vi "TeardownBeforeStart.vi"(6 "Error":errorcluster, 7 "ConcreteActor":refnum<class "ConcreteActor.lvclass">, 11 "UnheardMessages":refnum<class "Message.lvclass">[](array[class])) -> (5 "ConcreteActor":refnum<class "ConcreteActor.lvclass">)   [LabVIEW 2020, in "_Template.lvlib" / "ActorTemplate.lvlib" / "{{Name}}.lvlib" / "ConcreteActor.lvclass"]
uses:
  ConcreteActor.lvclass
  ConcreteActor.lvclass/ConcreteActor.ctl
  jettl/jettl/Actor/Actor.lvclass
  jettl/jettl/Message/Message.lvclass
panel:
  # "This front panel should not be manipulated."
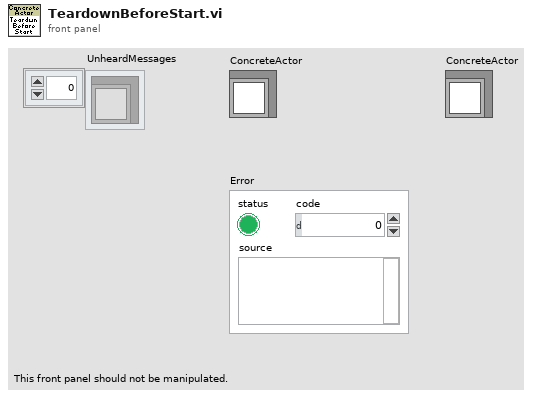
[diagram p1: front panel]
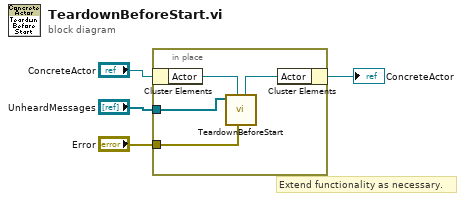
[diagram p0: block diagram]
diagram:
  # "Extend functionality as necessary."
  n1 = in-place {
    in-place-border: "UnheardMessages" -> [w6]
    in-place-border: "Error" -> [w5]
    n2 = in-place-cluster #1("ConcreteActor") -> ("Actor"=w8:refnum<class "Actor.lvclass">)
    n3 = call-dynamic "TeardownBeforeStart.vi"("Error"=w5, "Actor"=w8, "UnheardMessages"=w6) -> ("Actor"=w7:refnum<class "Actor.lvclass">)  [unwired: 8 in]
    n4 = in-place-cluster #1("Actor"=w7) -> (→"ConcreteActor":refnum<class "ConcreteActor.lvclass">)
  }
